vi "mqttCmdBuildPayload.vi"(0 "_mqtt in":refnum<class "mqttCmdSubscribe.lvclass">, 11 "error in (no error)":errorcluster) -> (4 "_mqtt out":refnum<class "mqttCmdSubscribe.lvclass">, 8 "payload":u8[](array[numeric]) format="%x", 15 "error out":errorcluster)   [LabVIEW 2021, in "mqttCmdSubscribe.lvclass"]
uses:
  mqttCmdSubscribe.lvclass
  mqttCmdSubscribe.lvclass/mqttCmdSubscribe.ctl
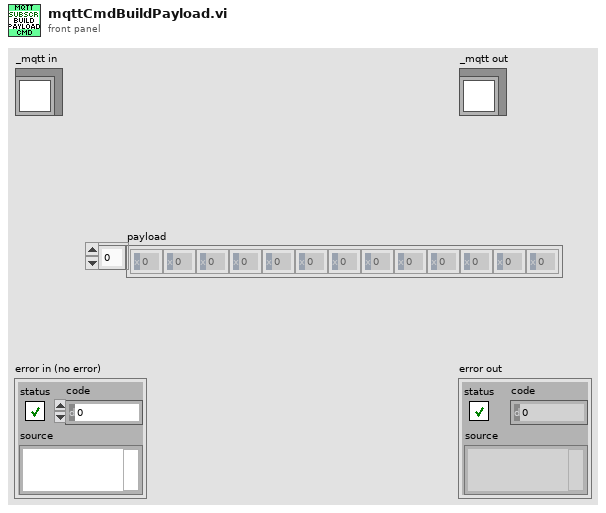
[diagram p1: front panel]
types:
  T1 = typedef "mqttSubscribeCluster.ctl" = cluster{"Topic":T2, "QoS":enum8{"At most once", "At least once", "Exactly once", "Reserved"}}
  T2 = typedef "Control 1.ctl" = string
  T3 = enum8{"At most once", "At least once", "Exactly once", "Reserved"}
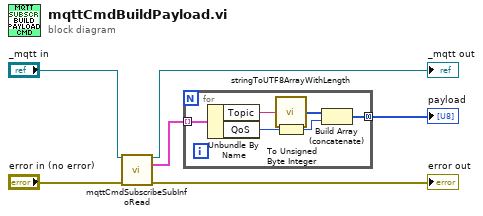
[diagram p0: block diagram]
diagram:
  n1 = call "mqttCmdSubscribeSubInfoRead.vi"("mqttSubscribe in"="_mqtt in", "error in (no error)"="error in (no error)") -> ("mqttSubscribe out"=→"_mqtt out":refnum<class "mqttCmdSubscribe.lvclass">, "subscriptionInfo"=w2:T1[], "error out"=→"error out":errorcluster)  [unwired: 11 in]
  n2 = for {
    tunnel: w2 -> [w12] mode=indexing
    tunnel: [w7] -> w6 mode=concatenating
    n3 = Unbundle By Name(w12) -> ("Topic"=w11:T2, "QoS"=w9:T3)
    n4 = call "stringToUTF8ArrayWithLength.vi"("string"=w11) -> ("UTF8[]"=w10:u8[])  [unwired: 14 in]
    n5 = To Unsigned Byte Integer(number=w9) -> (unsigned 8bit integer=w8:u8)
    n6 = Build Array (concatenate)(w10, w8) -> (w7:u8[])
  }
  "payload" <- w6
